vi "Fancy Light Controller.vi"(1 "error in":errorcluster) -> (0 "error out":errorcluster)   [LabVIEW 2017]
panel:
  out "Spark Input":dbl
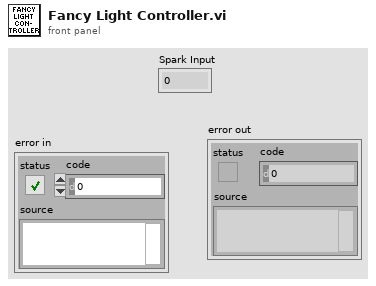
[diagram p1: front panel]
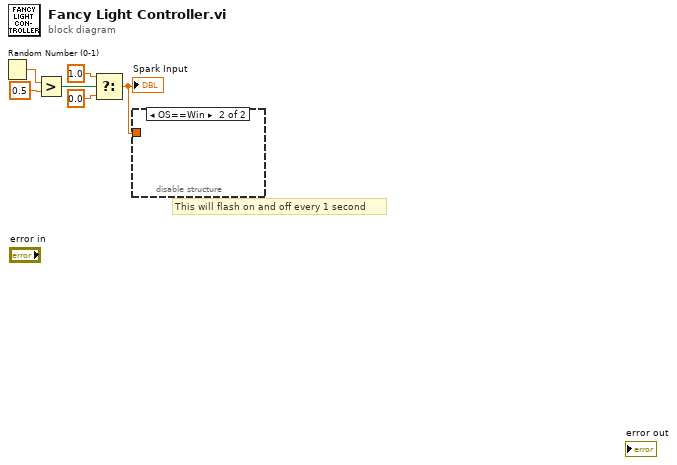
[diagram p0: block diagram]
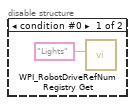
[diagram p2: hidden frame]
diagram:
  # "This will flash on and off every 1 second"
  n1 = Random Number (0-1)() -> (number: 0 to 1=w6:dbl)
  n2 = Greater?(x=w6, y=0.5) -> (0:w4:bool)
  n3 = Select(t=1.0, s=w4, f=0.0) -> (s? t:f=w1:dbl)
  "Spark Input" <- w1
  n4 = disable-structure shown="OS==Win" {
    disable-tunnel: w1 -> [_ _]
    frame condition #0 {
      n5 = call <vilib>:"WPI_RobotDriveRefNum Registry Get.vi"("refnum name"="Lights") -> ()  [unwired: 9 in, 2 out]
    }
    frame condition #1 (active) {
    }
  }
